vi "Read Core.vi"(8 "error in (no error)":errorcluster, 11 "WebView2.lvlib:WebView2 Control.lvclass":refnum<class "WebView2 Control.lvclass">) -> (0 "error out":errorcluster, 2 "Webview2 Core":refnum<k24>, 3 "WebView2.lvlib:WebView2 Control.lvclass":refnum<class "WebView2 Control.lvclass">)   [LabVIEW 2020, in "WebView2.lvlib" / "WebView2 Control.lvclass"]
uses:
  WebView2 Control.lvclass
  C:/Users/Simon/Documents/GitHub/LV-WebView2/Source/Libs/Microsoft.Web.WebView2.Core.dll
  Libs/Microsoft.Web.WebView2.Core.dll
  WebView2 Control.lvclass/WebView2 Control.ctl
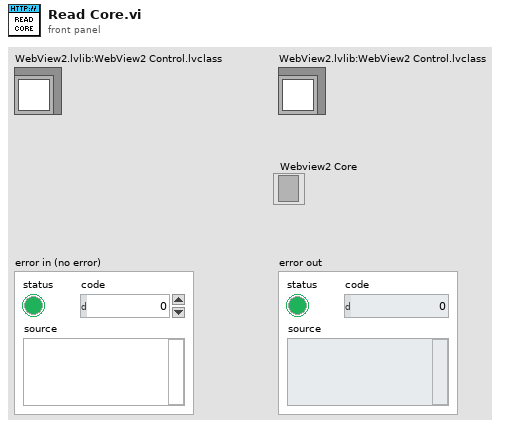
[diagram p1: front panel]
types:
  T1 = typedef "WebView2.lvlib/WebView2 Control.lvclass/Res.ctl" = cluster{"WebView2":refnum<k24>, "Webview2 Core":refnum<k24>, "event callback":refnum<k27>, "Environment":refnum<k24>}
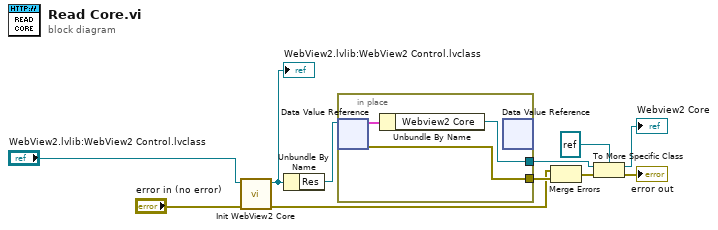
[diagram p0: block diagram]
diagram:
  n1 = call "Init WebView2 Core.vi"("error in (no error)"="error in (no error)", "WebView2"="WebView2.lvlib:WebView2 Control.lvclass") -> ("error out"=w5:errorcluster, "WebView2.lvlib:WebView2 Control.lvclass"=w7:refnum<class "WebView2 Control.lvclass">)  [unwired: 8 in]
  "WebView2.lvlib:WebView2 Control.lvclass" <- w7
  n2 = Unbundle By Name(w7) -> ("Res"=w9:refnum<data-value>)
  n3 = in-place {
    in-place-border: [w13] -> w3
    in-place-border: [w12] -> w11
    n4 = in-place-dvr #1(w9) -> (w14:T1, w12:errorcluster)
    n5 = Unbundle By Name(w14) -> ("Webview2 Core"=w13:refnum<k24>)
    n6 = in-place-dvr #1() -> ()  [unwired: 1 in, 2 out]
  }
  n7 = Merge Errors(w5, w11) -> (w10:errorcluster)
  n8 = To More Specific Class(target class=refnum<k24> refnum ("Webview2 Core"), reference=w3, error in=w10) -> (specific class reference=→"Webview2 Core":refnum<k24>, error out=→"error out":errorcluster)
